vi "Actor Core.vi"(8 "error in":errorcluster, 11 "Settings View in":refnum<class "Settings View.lvclass">) -> (0 "error out":errorcluster, 3 "Actor out":refnum<class "Actor.lvclass">)   [LabVIEW 2020, in "Settings View.lvlib" / "Settings View.lvclass"]
doc: "(<B>Filename</B>: Actor Framework.lvlib:Actor.lvclass:Actor Core.vi)\n\nReceives messages to the actor, reacts to them, and initiates any error handling that may shut the actor down.\n\nDescendant classes may override this VI to append parallel tasks for the actor to complete while it handles messages. Overrides use the Call Parent Method node."
uses:
  Settings View.lvclass
  C:/Program Files/National Instruments/LabVIEW 2020/vi.lib/ActorFramework/Actor/Actor.lvclass
  <vilib>/ActorFramework/Actor/Actor.lvclass
  <vilib>/ActorFramework/Actor/Actor.lvclass/Actor.ctl
  <vilib>/ActorFramework/Message Enqueuer/Message Enqueuer.lvclass/Message Enqueuer.ctl
  Settings View Messages/Broadcast Show Dialog Msg/Broadcast Show Dialog Msg.lvclass/Broadcast Show Dialog Msg.ctl
  <vilib>/ActorFramework/Message Enqueuer/Init from Existing Queue.vi
  <vilib>/ActorFramework/Message Enqueuer/Enqueue.vi
  Settings View Messages/Broadcast Show Dialog Msg/Broadcast Show Dialog Msg.lvclass
  C:/Program Files/National Instruments/LabVIEW 2020/vi.lib/ActorFramework/Message/Message.lvclass
  <vilib>/ActorFramework/Message Priority Queue/Priority Enqueue.vi
  <vilib>/ActorFrameworkMVC/Abstract View/Abstract View/Abstract View.lvclass
  <vilib>/ActorFramework/Message Enqueuer/Message Enqueuer.lvclass
panel:
  in  "Show Dialog Toggle Button":bool=TRUE
  # "Show exit dialog when close panel"
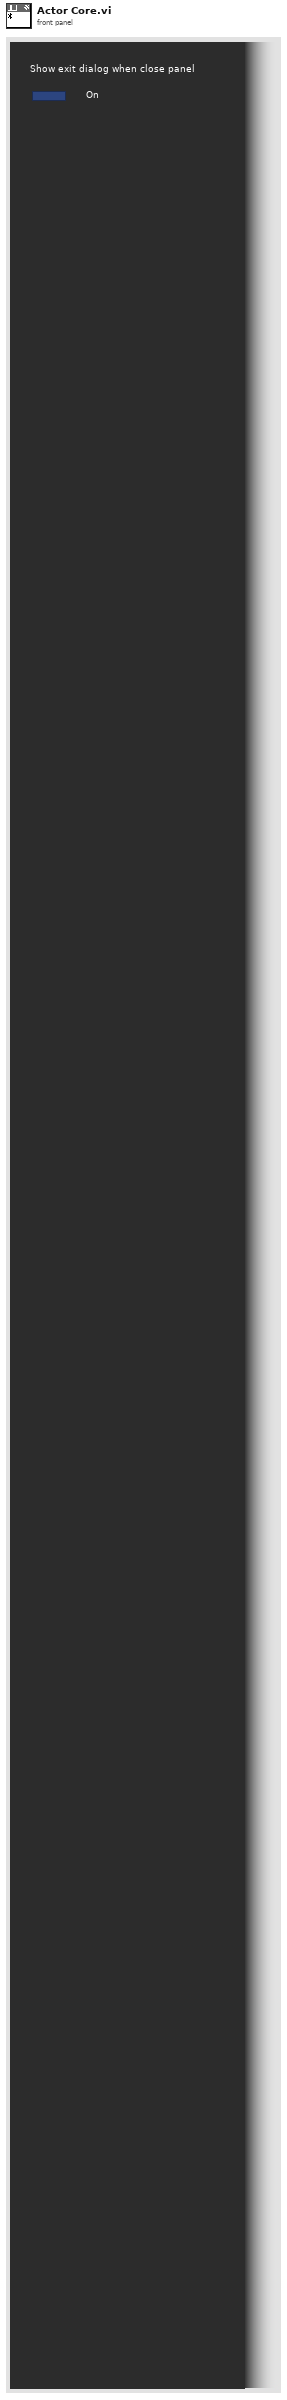
[diagram p1: front panel]
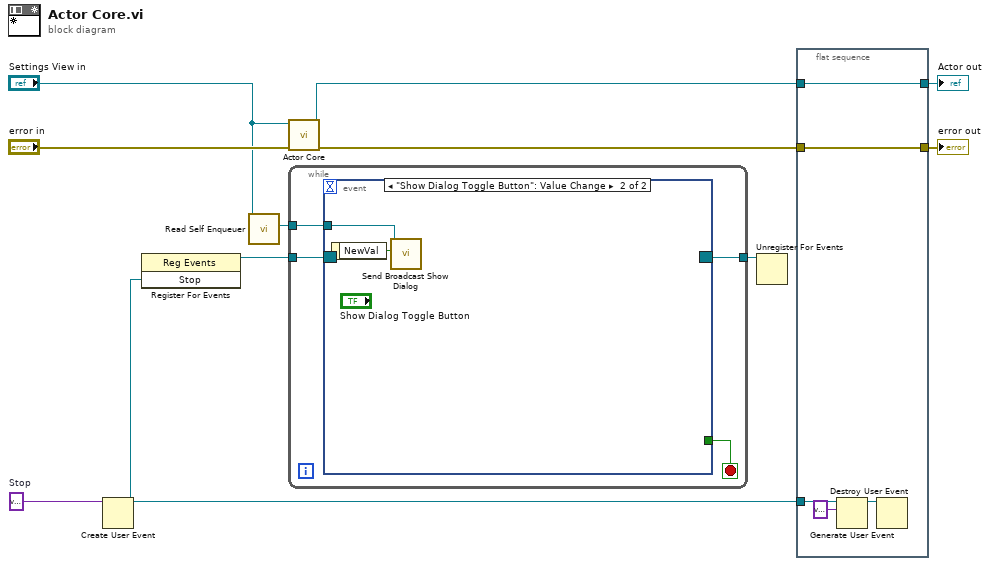
[diagram p0: block diagram]
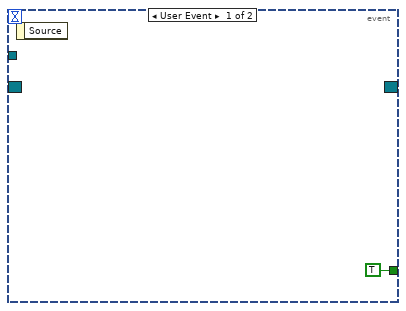
[diagram p2: hidden frame]
diagram:
  w9 = variant  # Stop
  n1 = Create User Event(user event datatype=w9) -> (user event=w3:refnum<user-event>)  [unwired: 1 in, 1 out]
  n2 = register-events(w3) -> (reference out=w10:refnum<event-registration>)  [unwired: 2 in, 1 out]
  n3 = call <vilib>:"Read Self Enqueuer.vi"("Actor"="Settings View in") -> ("Self Enqueuer"=w11:refnum<class "Message Enqueuer.lvclass">)  [unwired: 10 in]
  n4 = call-parent "Actor Core.vi"("error in"="error in", "Abstract View in"="Settings View in") -> ("error out"=w6:errorcluster, "Actor out"=w7:refnum<class "Actor.lvclass">)  [unwired: 8 in]
  n5 = while {
    tunnel: w11 -> [w12]
    tunnel: w10 -> [w15]
    tunnel: [w14] -> w8
    stop <- w13 stop-if-true
    n6 = event shown="[1] \"Show Dialog Toggle Button\": Value Change" {
      selector: w15 -> [_ _]
      dyn-events: [_ _] -> w14
      timeout: _ -> [_ _]
      tunnel: [TRUE _] -> w13
      tunnel: w12 -> [_ w18]
      event User Event {
        n7 = event-data() -> ()  [unwired: 1 in, 1 out]
      }
      event "Show Dialog Toggle Button": Value Change {
        n8 = event-data() -> ("NewVal"=w17:bool)  [unwired: 1 in]
        n9 = call "Send Broadcast Show Dialog.vi"("Show Dialog"=w17, "Message Enqueuer"=w18) -> ()  [unwired: 8 in, 2 out]
      }
    }
  }
  n10 = Unregister For Events(event registration refnum=w8) -> ()  [unwired: 1 in, 1 out]
  n11 = flat-sequence {
    tunnel: w3 -> [w23]
    tunnel: w7 -> [w20]
    tunnel: [w20] -> w2
    tunnel: w6 -> [w19]
    tunnel: [w19] -> w1
    frame #0 {
      n12 = Generate User Event(user event=w23, event data cluster=variant ("event data")) -> (user event out=w21:refnum<user-event>)  [unwired: 2 in, 1 out]
      n13 = Destroy User Event(user event=w21) -> ()  [unwired: 1 in, 1 out]
    }
  }
  "error out" <- w1
  "Actor out" <- w2
